vi "gsp_simulator_read_command.vi"(4 "error in (no error)":errorcluster) -> (0 "error out":errorcluster, 1 "Parameters":i32[](array[numeric]), 2 "Motor#":u8, 3 "Command#":u16)   [LabVIEW 2015]
uses:
  gsp_simulator_global.vi
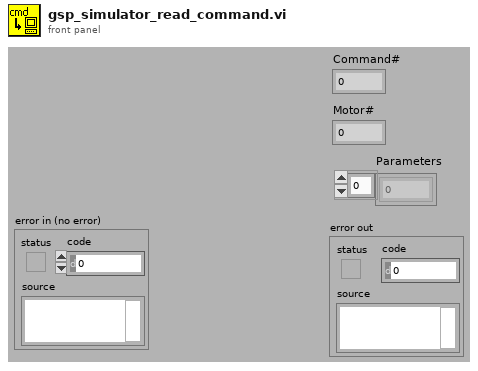
[diagram p1: front panel]
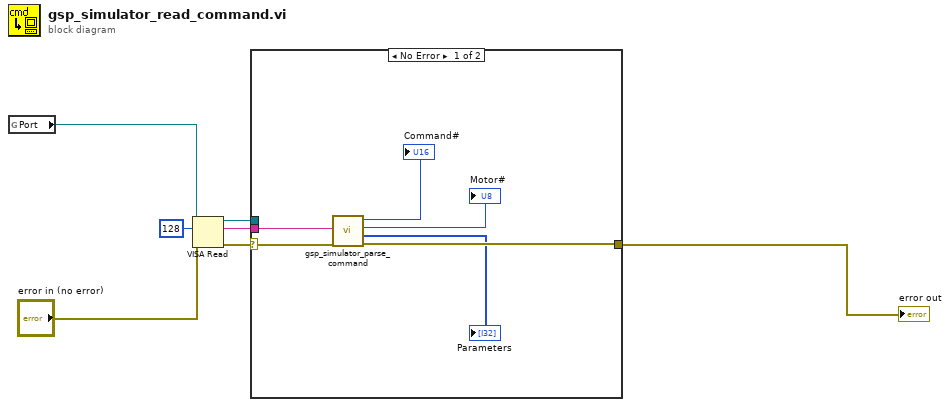
[diagram p0: block diagram]
diagram:
  n1 = global read "gsp_simulator_global.vi" "Port"() -> (w7:refnum<visa-resource-name>)
  n2 = VISA Read(VISA resource name=w7, byte count=u32 128, error in (no error)="error in (no error)") -> (VISA resource name out=w1:refnum<visa-resource-name>, read buffer=w2:string, error out=w4:errorcluster)  [unwired: 1 out]
  n3 = case shown="No Error" w4 {
    selector: w4 -> [w13 w14]
    tunnel: [w11 w14] -> w3
    tunnel: w2 -> [w12 _]
    tunnel: w1 -> [_ _]
    frame No Error {
      n4 = call "gsp_simulator_parse_command.vi"("error in (no error)"=w13, "commandstring"=w12) -> ("error out"=w11:errorcluster, "Parameters"=→"Parameters":i32[], "Motor#"=→"Motor#":u8, "Command#"=→"Command#":u16)  [unwired: 2 in]
    }
    frame Error {
    }
  }
  "error out" <- w3
